vi "Read Name core.vi"(11 "Close VIPM Step in":refnum<class "Close VIPM Step.lvclass">) -> (2 "Name":string)   [LabVIEW 2019, in "VIPM.lvlib" / "Close VIPM Step.lvclass"]
doc: "Gets the name for the build step\n\nCopyright: MGI 2016\nAuthor: Derek Trepanier"
uses:
  Close VIPM Step.lvclass
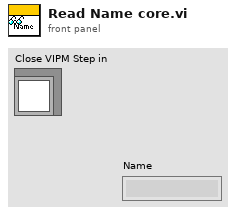
[diagram p1: front panel]
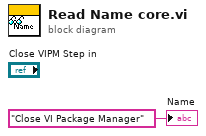
[diagram p0: block diagram]
diagram:
  "Name" <- "Close VI Package Manager" ("Name")
